vi "Main_control_system.vi"(0 "read buffer":string, 5 "Measurement in":dbl, 7 "Numeric":i32, 9 "Measurement channel 2":dbl, 11 "Max. Load Current":dbl=-0.5 format="%#_13g") -> (4 "Action":string, 6 "Measurement out":dbl)   [LabVIEW 2015]
uses:
  utilities/Test_Code/Global 5.vi
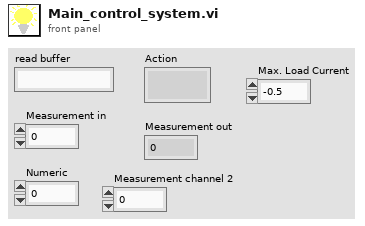
[diagram p1: front panel]
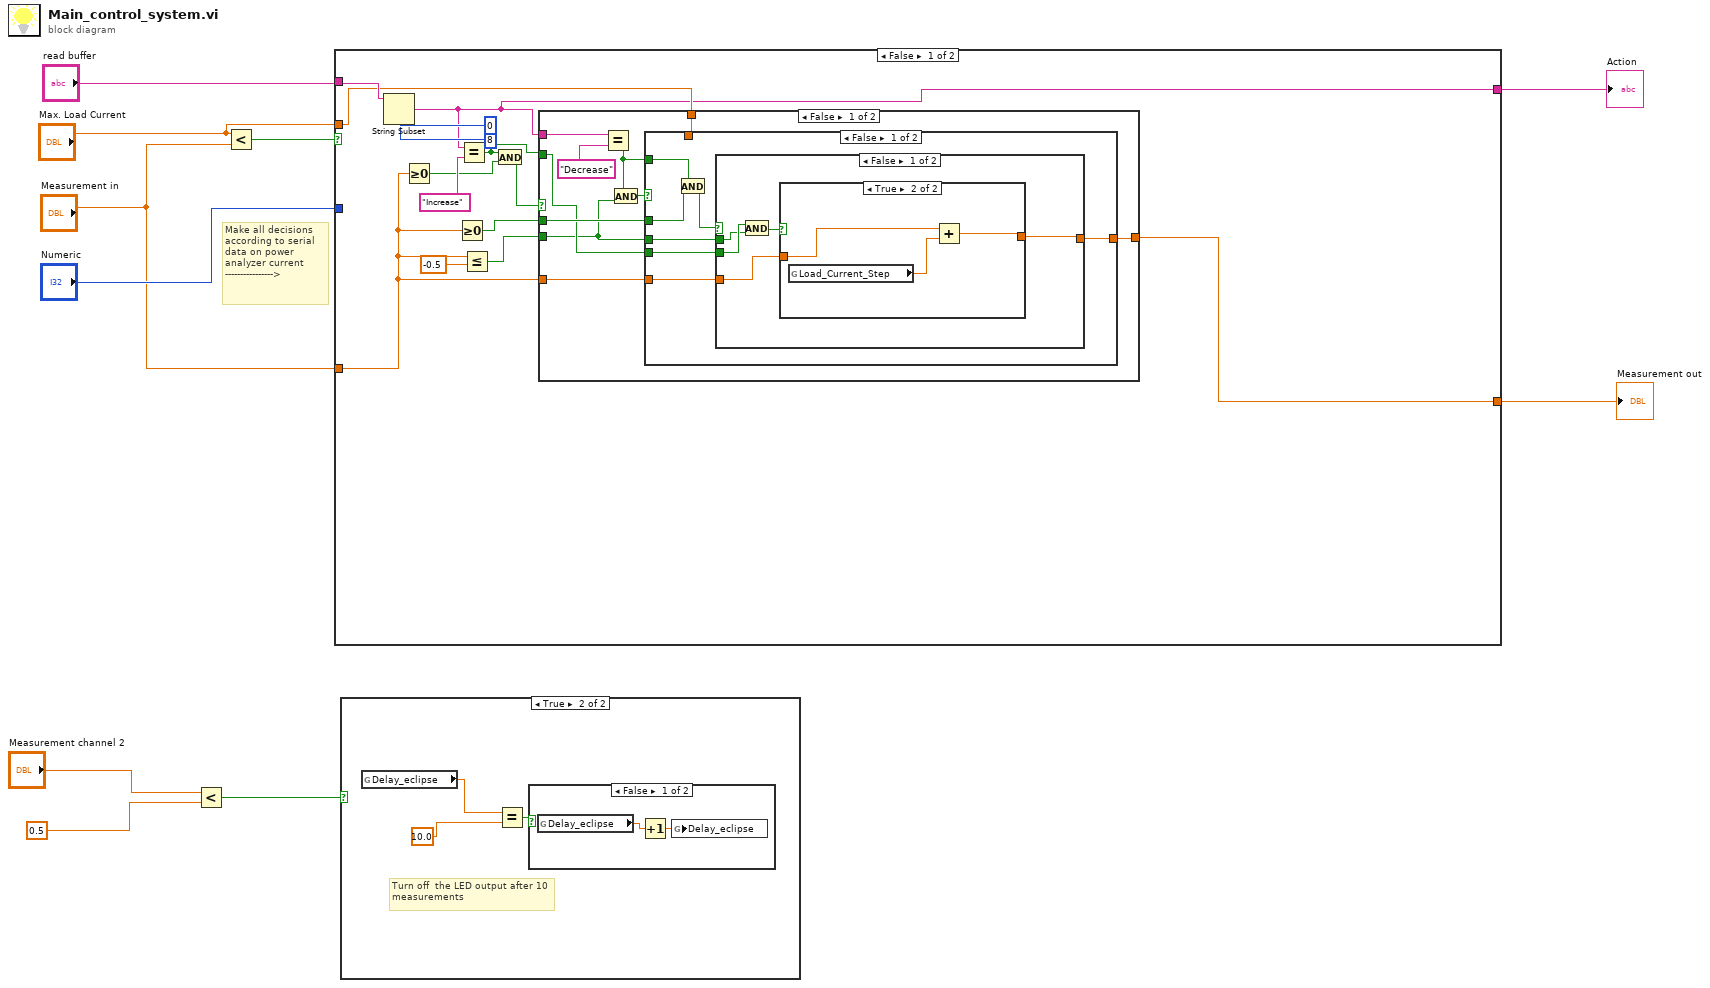
[diagram p0: block diagram]
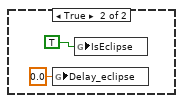
[diagram p3: hidden frame]
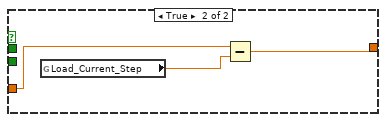
[diagram p5: hidden frame]
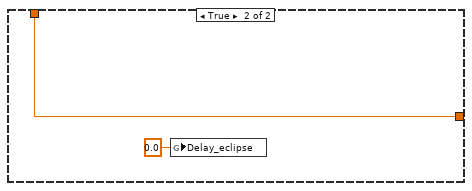
[diagram p6: hidden frame]
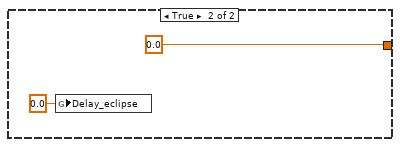
[diagram p7: hidden frame]
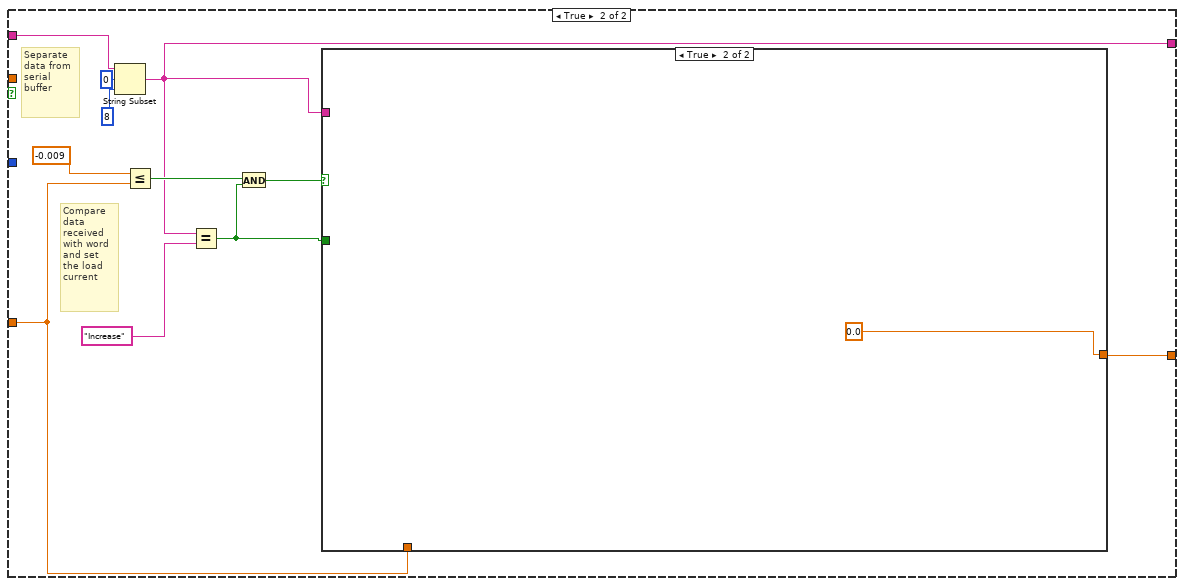
[diagram p8: hidden frame]
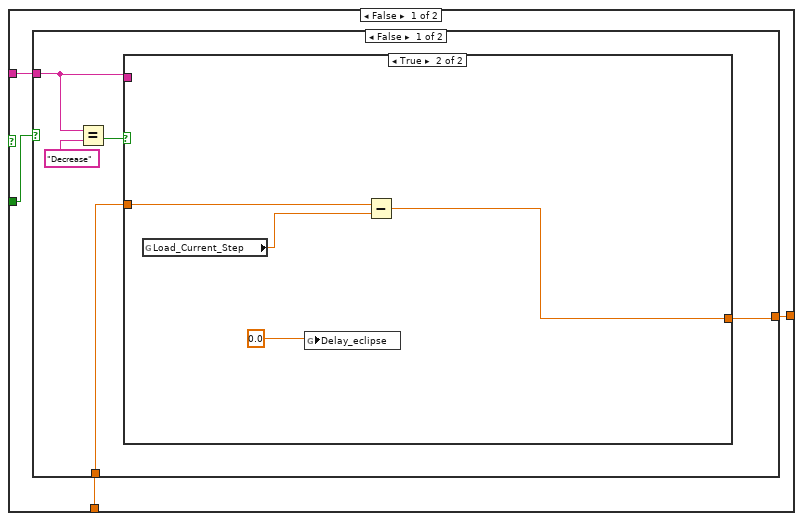
[diagram p9: hidden frame]
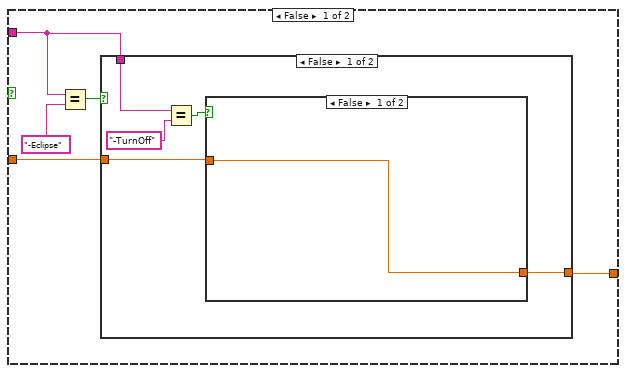
[diagram p10: hidden frame]
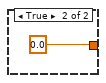
[diagram p11: hidden frame]
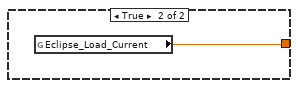
[diagram p12: hidden frame]
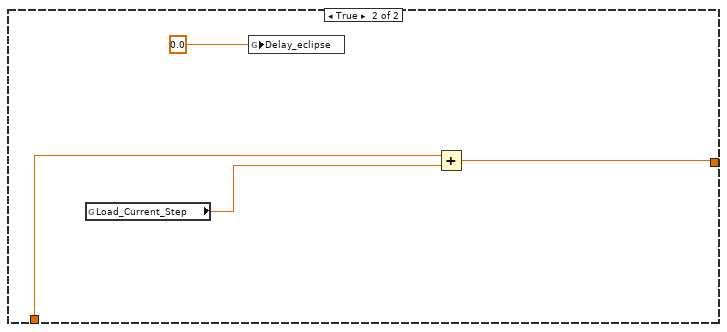
[diagram p13: hidden frame]
diagram:
  # "Make all decisions according to serial data on power analyzer current\n---------------->"
  n1 = Less?(x="Measurement channel 2", y=0.5) -> (x < y?=w3:bool)
  n2 = Less?(x="Max. Load Current", y="Measurement in") -> (x < y?=w6:bool)
  n3 = case shown="False" w6 {
    tunnel: [w24 w68] -> w10
    tunnel: "Measurement in" -> [w14 w62]
    tunnel: "read buffer" -> [w17 w66]
    tunnel: "Numeric" -> [_ _]
    tunnel: "Max. Load Current" -> [w12 _]
    tunnel: [w11 w58] -> w4
    frame False {
      n4 = String Subset(string=w17, offset (0)=0, length (rest)=8 ("length (rest)")) -> (substring=w11:string)
      n5 = Greater Or Equal To 0?(x=w14) -> (x >= 0?=w13:bool)
      n6 = Greater Or Equal To 0?(x=w14) -> (x >= 0?=w16:bool)
      n7 = Equal?(x=w11, y="Increase") -> (x = y?=w15:bool)
      n8 = Less Or Equal?(x=w14, y=-0.5) -> (x <= y?=w21:bool)
      n9 = And(x=w15, y=w13) -> (x .and. y?=w23:bool)
      n10 = case shown="False" w23 {
        tunnel: [w31 0.0] -> w24
        tunnel: w21 -> [w26 _]
        tunnel: w11 -> [w33 _]
        tunnel: w16 -> [w29 _]
        tunnel: w14 -> [w28 _]
        tunnel: w15 -> [w27 _]
        tunnel: w12 -> [w25 _]
        frame False {
          n11 = Equal?(x=w33, y="Decrease") -> (x = y?=w30:bool)
          n12 = And(x=w30, y=w26) -> (x .and. y?=w34:bool)
          n13 = case shown="False" w34 {
            tunnel: [w38 w55] -> w31
            tunnel: w30 -> [w40 _]
            tunnel: w29 -> [w39 _]
            tunnel: w28 -> [w37 _]
            tunnel: w27 -> [w36 _]
            tunnel: w26 -> [w35 _]
            tunnel: w25 -> [_ w55]
            frame False {
              n14 = And(x=w40, y=w39) -> (x .and. y?=w41:bool)
              n15 = case shown="False" w41 {
                tunnel: [w43 w53] -> w38
                tunnel: w37 -> [w42 w52]
                tunnel: w36 -> [w46 _]
                tunnel: w35 -> [w45 _]
                frame False {
                  n16 = And(x=w46, y=w45) -> (x .and. y?=w44:bool)
                  n17 = case shown="True" w44 {
                    tunnel: [w47 w50] -> w43
                    tunnel: w42 -> [w47 w49]
                    frame False {
                    }
                    frame True {
                      n18 = global read "Global 5.vi" "Load_Current_Step"() -> (w48:dbl)
                      n19 = Add(x=w49, y=w48) -> (x+y=w50:dbl)
                    }
                  }
                }
                frame True {
                  n20 = global read "Global 5.vi" "Load_Current_Step"() -> (w51:dbl)
                  n21 = Subtract(x=w52, y=w51) -> (x-y=w53:dbl)
                }
              }
            }
            frame True {
              n22 = global write "Global 5.vi" "Delay_eclipse"(0.0 ("Delay_eclipse")) -> ()
            }
          }
        }
        frame True {
          n23 = global write "Global 5.vi" "Delay_eclipse"(0.0 ("Delay_eclipse")) -> ()
        }
      }
    }
    frame True {
      # "Compare data received with word and set the load current"
      # "Separate data from serial buffer"
      n24 = String Subset(string=w66, offset (0)=0, length (rest)=8 ("length (rest)")) -> (substring=w58:string)
      n25 = Less Or Equal?(x=-0.009, y=w62) -> (x <= y?=w59:bool)
      n26 = Equal?(x=w58, y="Increase") -> (x = y?=w61:bool)
      n27 = And(x=w59, y=w61) -> (x .and. y?=w60:bool)
      n28 = case shown="True" w60 {
        tunnel: [w72 0.0 ("Measurement")] -> w68
        tunnel: w61 -> [w71 _]
        tunnel: w62 -> [w70 _]
        tunnel: w58 -> [w69 _]
        frame False {
          n29 = case shown="False" w71 {
            tunnel: [w77 w98] -> w72
            tunnel: w69 -> [w73 _]
            tunnel: w70 -> [w74 w97]
            frame False {
              n30 = Equal?(x=w73, y="Decrease") -> (x = y?=w76:bool)
              n31 = case shown="True" w76 {
                tunnel: [w80 w94] -> w77
                tunnel: w74 -> [w79 w93]
                tunnel: w73 -> [w78 _]
                frame False {
                  n32 = Equal?(x=w78, y="-Eclipse") -> (x = y?=w82:bool)
                  n33 = case shown="False" w82 {
                    tunnel: [w84 w90] -> w80
                    tunnel: w79 -> [w83 _]
                    tunnel: w78 -> [w86 _]
                    frame False {
                      n34 = Equal?(x=w86, y="-TurnOff") -> (x = y?=w87:bool)
                      n35 = case shown="False" w87 {
                        tunnel: [w88 0.0 ("x")] -> w84
                        tunnel: w83 -> [w88 _]
                        frame False {
                        }
                        frame True {
                        }
                      }
                    }
                    frame True {
                      n36 = global read "Global 5.vi" "Eclipse_Load_Current"() -> (w90:dbl)
                    }
                  }
                }
                frame True {
                  n37 = global read "Global 5.vi" "Load_Current_Step"() -> (w92:dbl)
                  n38 = global write "Global 5.vi" "Delay_eclipse"(0.0 ("Delay_eclipse")) -> ()
                  n39 = Subtract(x=w93, y=w92) -> (x-y=w94:dbl)
                }
              }
            }
            frame True {
              n40 = global read "Global 5.vi" "Load_Current_Step"() -> (w96:dbl)
              n41 = global write "Global 5.vi" "Delay_eclipse"(0.0 ("Delay_eclipse")) -> ()
              n42 = Add(x=w97, y=w96) -> (x+y=w98:dbl)
            }
          }
        }
        frame True {
        }
      }
    }
  }
  "Measurement out" <- w10
  "Action" <- w4
  n43 = case shown="True" w3 {
    frame False {
    }
    frame True {
      # "Turn off  the LED output after 10 measurements"
      n44 = global read "Global 5.vi" "Delay_eclipse"() -> (w102:dbl)
      n45 = Equal?(x=w102, y=10.0) -> (x = y?=w100:bool)
      n46 = case shown="False" w100 {
        frame False {
          n47 = global read "Global 5.vi" "Delay_eclipse"() -> (w103:dbl)
          n48 = Increment(x=w103) -> (x+1=w104:dbl)
          n49 = global write "Global 5.vi" "Delay_eclipse"(w104) -> ()
        }
        frame True {
          n50 = global write "Global 5.vi" "Delay_eclipse"(0.0 ("i")) -> ()
          n51 = global write "Global 5.vi" "IsEclipse"(TRUE ("Boolean")) -> ()
        }
      }
    }
  }
